vi "uPythonApp.vi"() -> ()   [LabVIEW 2019]
uses:
  <userlib>/MicroPython/VIs/uPythonX/uPythonX.xctl
panel:
  in  "uPythonX":T1(xcontrol)={"VISA Refnum in"="", "All Code"="'''\nGetting Started with MicroPython\nWelcome to MicroPython - a subset of python for small microprocessors.  \nTo get started, make sure your Spike is on, you are connected in one of\n the three ways (Terminal, Python, or LabVIEW) and try running this code:\n'''\nimport hub\nhub.display.show(‘Tufts’)\n\n'''\nNotice the “import” command - that pulls in a python library that lets you talk to Spike.  \nOne of the more powerful attributes of Python is that you can test anything out before \nwriting code in the REPL (read eval print loop).  It will execute any python command - \ntry typing 2 + 2 below and see what it says:\n     \n>>> 2 + 2\n\nnow try typing hub.display(‘your name’) - note that since you already imported hub above, \nit is already in memory.  If it were not, you would get an error like:\n\nTraceback…..\n\nNow it is time to explore.  Hub has a lot of functions - you can find out by looking \nat the documentation here or by just typing hub. and then hitting the TAB key in \nthe REPL.  That will show you all the different ways you can complete the command.  \nSee if you can read the acceleration.\n\nThe acceleration comes back as an array of values - so if you just want the X value, \nyou can try hub.motion.accelerometer()[0] or nicer code would be to use variables like this:\n'''\nimport hub\n\naccel = hub.motion.accelerometer()\nxAccel = accel[0]\nhub.display.show(str(xAccel))\n'''\nYou could also display all three accelerations using a loop.  We will also import the \nlibrary utime so that we can pause and give you time to read the number on the screen.  \nTry this code:\n'''\nimport hub,utime\n\naccel = hub.motion.accelerometer()\nfor Acc in accel:\n     hub.display.show(str(Acc))\n     utime.sleep(0.8)\n'''\nAt this point a few things become important:\nspaces - Python is all about indenting right - similar to brackets in other languages,\n indentation tells you what is inside the for loop and what is not.  When using the REPL, \n you will notice that when you indent, it no longer executes the line but rather \n waits for you to finish the lines for the for loop before executing (and the >>> \nis replaced by …).  To finish the for loop, just hit return three times and the loop will be executed.\n\nNext, see if you can figure out what the code below does - and try executing it to see if \nyou are right.  Hint -you need a sensor on port B.\n'''\nimport hub,utime\n\nwhile True:\n     accel = hub.motion.accelerometer()\n     for Acc in accel:\n         hub.display.show(str(Acc))\n          utime.sleep(0.8)\n     if hub.port.B.device.get():\n         break"}
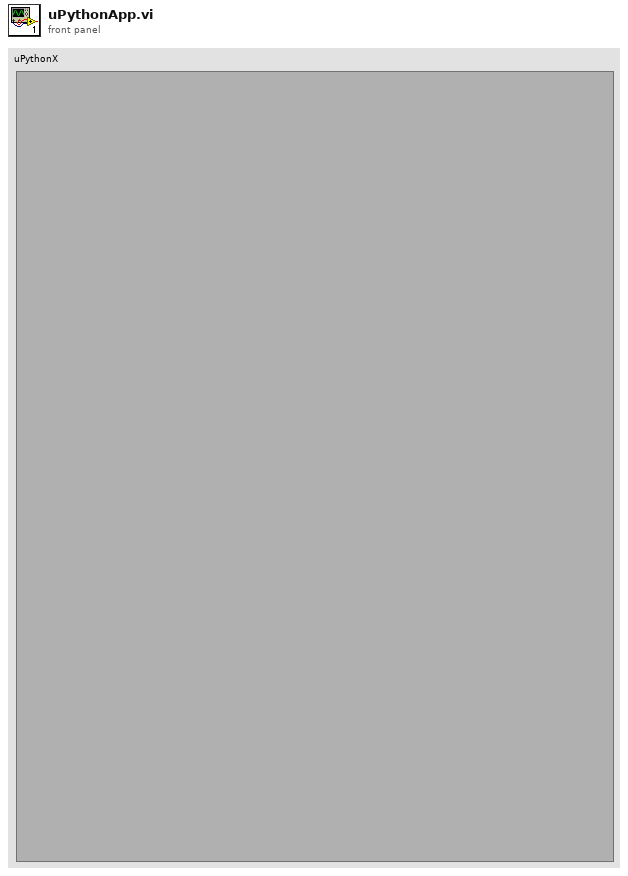
[diagram p1: front panel]
types:
  T1 = cluster{"VISA Refnum in":refnum<visa-resource-name>, "All Code":string}
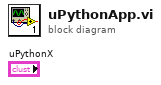
[diagram p0: block diagram]
diagram:
